vi "Compute Traffic Heat Map.vi"(8 "error in (no error)":errorcluster, 11 "TrafficMap in":refnum<class "TrafficMap.lvclass">) -> (0 "error out":errorcluster, 2 "Traffic Map":u32[][](graph), 3 "TrafficMap out":refnum<class "TrafficMap.lvclass">)   [LabVIEW 2017, in "TrafficMap.lvclass"]
uses:
  TrafficMap.lvclass
  TrafficMap.lvclass/TrafficMap.ctl
  Zone/Zone.lvclass/Zone.ctl
  Zone/Zone.lvclass
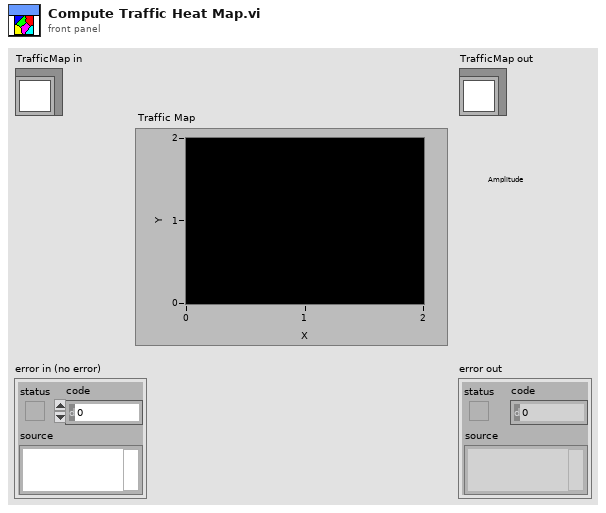
[diagram p1: front panel]
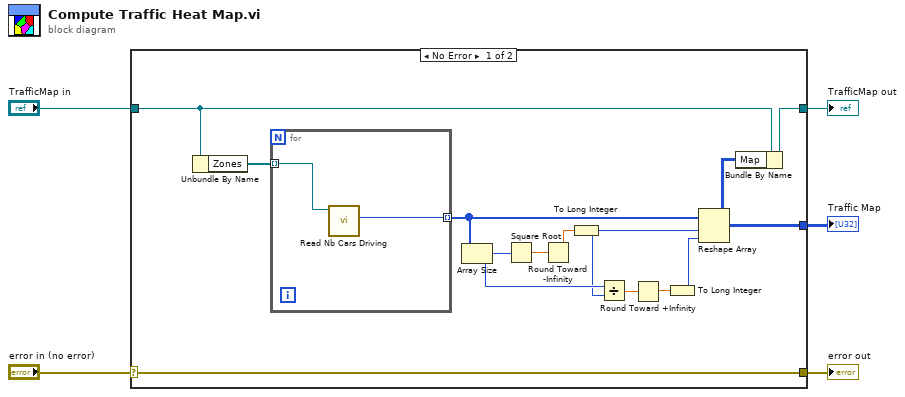
[diagram p0: block diagram]
diagram:
  n1 = case shown="No Error" "error in (no error)" {
    selector: "error in (no error)" -> [w18 w22]
    tunnel: [w18 w22] -> w4
    tunnel: [w7 w21] -> w2
    tunnel: "TrafficMap in" -> [w8 w21]
    tunnel: [w6 _] -> w1
    frame No Error {
      n2 = Unbundle By Name(w8) -> ("Zones"=w17:refnum<class "Zone.lvclass">[])
      n3 = for {
        tunnel: w17 -> [w20] mode=indexing
        tunnel: [w19] -> w16 mode=indexing
        n4 = call "Read Nb Cars Driving.vi"("Zone in"=w20) -> ("Nb Cars Driving"=w19:u32)  [unwired: 8 in, 2 out]
      }
      n5 = Array Size(array=w16) -> (size(s)=w13:i32)
      n6 = Square Root(x=w13) -> (sqrt(x)=w15:dbl)
      n7 = Round Toward -Infinity(1:w15) -> (0:w14:dbl)
      n8 = To Long Integer(number=w14) -> (32bit integer=w12:i32)
      n9 = Divide(x=w13, y=w12) -> (x/y=w11:dbl)
      n10 = Round Toward +Infinity(x=w11) -> (ceil(x): smallest int >= x=w10:dbl)
      n11 = To Long Integer(number=w10) -> (32bit integer=w9:i32)
      n12 = Reshape Array(w16, w12, w9) -> (w6:u32[][])
      n13 = Bundle By Name(cluster=w8, "Map"=w6) -> (w7:refnum<class "TrafficMap.lvclass">)
    }
    frame Error {
    }
  }
  "error out" <- w4
  "TrafficMap out" <- w2
  "Traffic Map" <- w1
